vi "niRFUtil RFHS FIFO Read.vi"(0 "Fifo ID":T1, 5 "Samples":i32=30720, 11 "error in (no error)":errorcluster) -> (4 "Fifo ID (out)":T1, 6 "IQ Samples (out)":csg[](array[numeric]), 15 "error out":errorcluster)   [LabVIEW 2015, in "niRFUtil.lvlib"]
uses:
  niRFUtil.lvlib
  niRFUtil RFHS FIFO Reference.ctl
  niRFUtil RFHS FIFO.ctl
  niRFUtil RFHS FIFO Error Codes.ctl
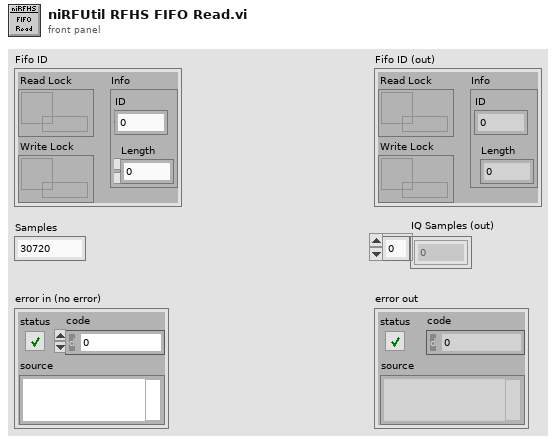
[diagram p1: front panel]
types:
  T1 = typedef "niRFUtil.lvlib/niRFUtil RFHS FIFO Reference.ctl" = cluster{"Read Lock":refnum<data-value>, "Info":T2, "Write Lock":refnum<data-value>}
  T2 = typedef "niRFUtil.lvlib/niRFUtil RFHS FIFO.ctl" = cluster{"ID":u64, "Length":u32}
  T3 = typedef "niRFUtil.lvlib/niRFUtil RFHS FIFO Error Codes.ctl" = i32
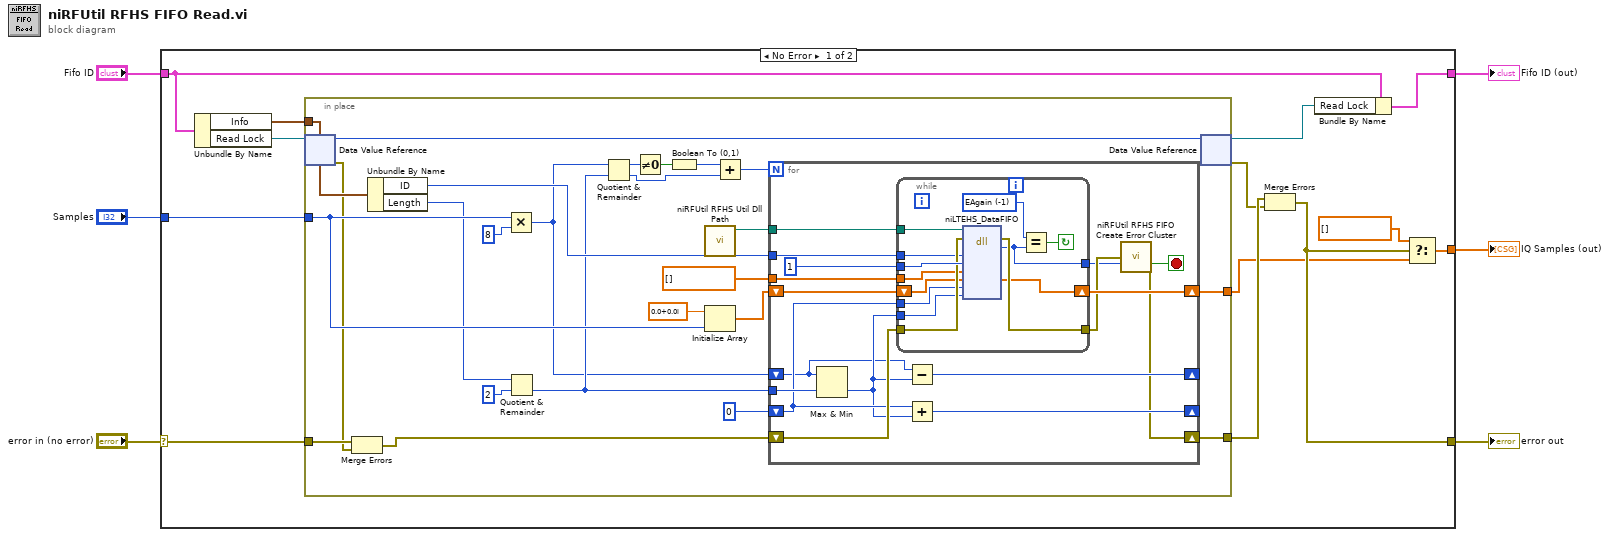
[diagram p0: block diagram]
diagram:
  n1 = case shown="No Error" "error in (no error)" {
    selector: "error in (no error)" -> [w19 w75]
    tunnel: "Samples" -> [w18 _]
    tunnel: [w10 _] -> w4
    tunnel: [w11 w75] -> w3
    tunnel: "Fifo ID" -> [w15 w74]
    tunnel: [w13 w74] -> w1
    frame No Error {
      n2 = Unbundle By Name(w15) -> ("Info"=w16:T2, "Read Lock"=w17:refnum<data-value>)
      n3 = in-place {
        in-place-border: w19 -> [w24]
        in-place-border: [w43] -> w12
        in-place-border: [w42] -> w9
        in-place-border: w18 -> [w41]
        in-place-border: w16 -> [w26]
        n4 = in-place-dvr #1(w17) -> (w25:i32, w22:errorcluster)
        n5 = Merge Errors(w24, w22) -> (w23:errorcluster)
        n6 = Unbundle By Name(w26) -> ("ID"=w35:u64, "Length"=w34:u32)
        n7 = Multiply(x=w41, y=8) -> (x*y=w20:i32)
        n8 = Quotient & Remainder(x=w34, y=u32 2) -> (floor(x/y)=w27:u32)  [unwired: 1 out]
        n9 = Quotient & Remainder(x=w20, y=w27) -> (x-y*floor(x/y)=w33:u32, floor(x/y)=w30:u32)
        n10 = Not Equal To 0?(x=w33) -> (x != 0?=w32:bool)
        n11 = Boolean To (0,1)(Boolean=w32) -> (0, 1=w31:i16)
        n12 = call "niRFUtil RFHS Util Dll Path.vi"() -> ("Path"=w36:path)  [unwired: 7 in, 4 out]
        n13 = Initialize Array(csg 0.0+0.0i ("Numeric"), w41) -> (w37:csg[])
        n14 = Add(x=w31, y=w30) -> (x+y=w29:u32)
        n15 = for {
          N: w29 -> [_]
          tunnel: csg[] [] ("IQ Samples") -> [w58]
          tunnel: w36 -> [w56]
          tunnel: w35 -> [w55]
          shift-right: [w47] -> w43
          shift-left: w23 -> [w59]
          shift-right: [w54] -> w42
          shift-left: w37 -> [w57]
          shift-right: [w49] -> _
          shift-left: u32 0 -> [w51]
          tunnel: w27 -> [w53]
          shift-right: [w52] -> _
          shift-left: w20 -> [w44]
          stop <- w45 stop-if-true
          n16 = Max & Min(x=w44, y=w53) -> (min(x,y)=w50:u32)  [unwired: 1 out]
          n17 = while {
            tunnel: u32 1 ("what") -> [w73]
            tunnel: w59 -> [w72]
            tunnel: [w71] -> w48
            tunnel: w58 -> [w70]
            tunnel: w56 -> [w67]
            tunnel: w55 -> [w66]
            shift-right: [w68] -> w54
            shift-left: w57 -> [w69]
            tunnel: w51 -> [w65]
            tunnel: w50 -> [w64]
            tunnel: [w61] -> w46
            stop <- w63 continue-if-true
            w62 = T3 -1 items=["OK"=1, "EAgain"=-1, "EZombie"=-2] ("Fifo error states")
            n18 = dll-call lib="M:/RfProtocols/RFmx/DLLs/niRFHS/trunk/2.0/dist/win32U/niRFHS_generic.dll" fn="niLTEHS_DataFIFO"(path in=w67, error in=w72, "fifoID"=w66, "what"=w73, "iBuf"=w70, "oBuf"=w69, "offset"=w65, "bytes"=w64) -> (error out=w71:errorcluster, "return type"=w61:i32, "oBuf"=w68:csg[])  [unwired: 6 in, 1 out]
            n19 = Equal?(x=w62, y=w61) -> (x = y?=w63:bool)
          }
          n20 = Subtract(x=w44, y=w50) -> (x-y=w52:u32)
          n21 = Add(x=w51, y=w50) -> (x+y=w49:u32)
          n22 = call "niRFUtil RFHS FIFO Create Error Cluster.vi"("error in (no error)"=w48, "fifo return value"=w46) -> ("error  out"=w47:errorcluster, "is error?"=w45:bool)  [unwired: 12 in]
        }
        n23 = in-place-dvr #1(w25) -> (w14:refnum<data-value>, w7:errorcluster)
      }
      n24 = Merge Errors(w12, w7) -> (w11:errorcluster)
      n25 = Bundle By Name(cluster=w15, "Read Lock"=w14) -> (w13:T1)
      n26 = Select(t=csg[] [] ("IQ Samples"), s=w11, f=w9) -> (s? t:f=w10:csg[])
    }
    frame Error {
    }
  }
  "error out" <- w3
  "IQ Samples (out)" <- w4
  "Fifo ID (out)" <- w1
